vi "Reset_DAQ.vi"(8 "error in (no error)":errorcluster) -> (0 "error out":errorcluster)   [LabVIEW 2017]
doc: "This VI resets all DAQ devices of a current hardware configuration, i.e. all detected devices in NI MAX."
uses:
  <vilib>/DAQmx/write.llb/DAQmx Write (Analog DBL 1Chan 1Samp).vi
  <vilib>/DAQmx/create/channels.llb/DAQmx Create Channel (AO-Voltage-Basic).vi
  <vilib>/DAQmx/miscellaneous.llb/DAQmx Fill In Error Info.vi
  <resource>/objmgr/daqmx.rc
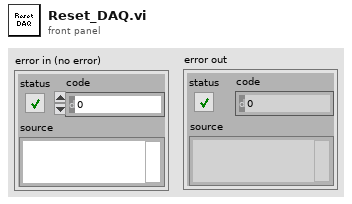
[diagram p1: front panel]
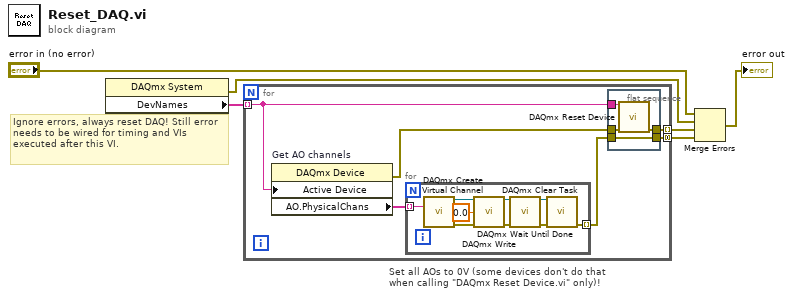
[diagram p0: block diagram]
diagram:
  # "Ignore errors, always reset DAQ! Still error needs to be wired for timing and VIs executed after this VI."
  n1 = property class="DAQmx System"() -> (error out=w2:errorcluster, "DevNames"=w6:tag[])  [unwired: 2 in, 1 out]
  n2 = for {
    tunnel: w6 -> [w11] mode=indexing
    tunnel: [w12] -> w5 mode=indexing
    tunnel: [w7] -> w1 mode=concatenating
    n3 = property on="Get AO channels" class="DAQmx Device"("Active Device"=w11) -> (error out=w9:errorcluster, "AO.PhysicalChans"=w10:tag[])  [unwired: 2 in, 1 out]
    n4 = for "Set all AOs to 0V (some devices don't do that when calling \"DAQmx Reset Device.vi\" only)!" {
      tunnel: w10 -> [w25] mode=indexing
      tunnel: [w17] -> w8 mode=indexing
      n5 = call-poly <vilib>:"DAQmx Create Virtual Channel.vi"("physical channels"=w25) -> ("task out"=w22:refnum<k21>, "error out"=w23:errorcluster)  [unwired: 13 in]
      n6 = call-poly <vilib>:"DAQmx Write.vi"("task/channels in"=w22, "data"=0.0, "error in"=w23) -> ("task out"=w20:refnum<k21>, "error out"=w21:errorcluster)  [unwired: 10 in, 1 out]
      n7 = call <vilib>:"DAQmx Wait Until Done.vi"("task/channels in"=w20, "error in"=w21) -> ("task out"=w18:refnum<k21>, "error out"=w19:errorcluster)  [unwired: 12 in]
      n8 = call <vilib>:"DAQmx Clear Task.vi"("task in"=w18, "error in"=w19) -> ("error out"=w17:errorcluster)  [unwired: 13 in]
    }
    n9 = flat-sequence {
      tunnel: [w16] -> w12
      tunnel: w11 -> [w15]
      tunnel: w9 -> [w14]
      tunnel: w8 -> [w13]
      tunnel: [w13] -> w7
      frame #0 {
        n10 = call <vilib>:"DAQmx Reset Device.vi"("device in"=w15, "error in"=w14) -> ("error out"=w16:errorcluster)  [unwired: 13 in]
      }
    }
  }
  n11 = Merge Errors("error in (no error)", w2, w5, w1) -> (→"error out":errorcluster)
